vi "EL2008.vi"(8 "error in (no error)":errorcluster, 11 "EL2008 Channels":T1) -> (0 "error out":errorcluster, 3 "Read Status":bool[](array[boolean]), 7 "Write Status":bool[](array[boolean]))   [LabVIEW 2022 SP3, in "IO_Library.lvlib"]
doc: "VI implementing the EL2008.\n\nBlock reads and writes to a terminal.\n\nTo use, modify the constant string entering the ADS Init block with your string (created with the ADS Path Helper)."
uses:
  IO_Library.lvlib
  TypeDefs/EL2008Outputs.ctl
  ADS/ADS_Library.lvlib
panel:
  out "EL2008 Wc State":variant[](array[variant])
  out "bHasMatched":bool[](array[boolean])
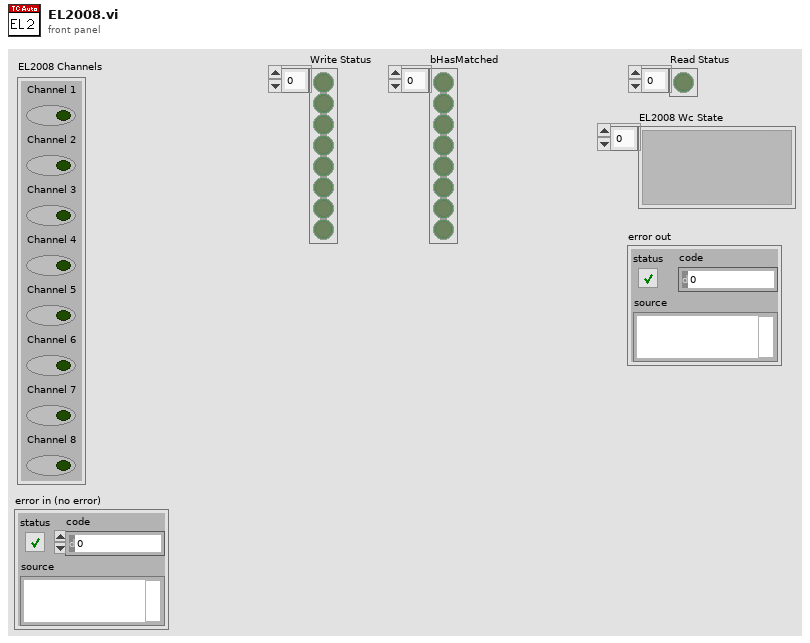
[diagram p1: front panel]
types:
  T1 = typedef "IO_Library.lvlib/EL2008Outputs.ctl" = cluster{"Channel 1":bool, "Channel 2":bool, "Channel 3":bool, "Channel 4":bool, "Channel 5":bool, "Channel 6":bool, "Channel 7":bool, "Channel 8":bool}
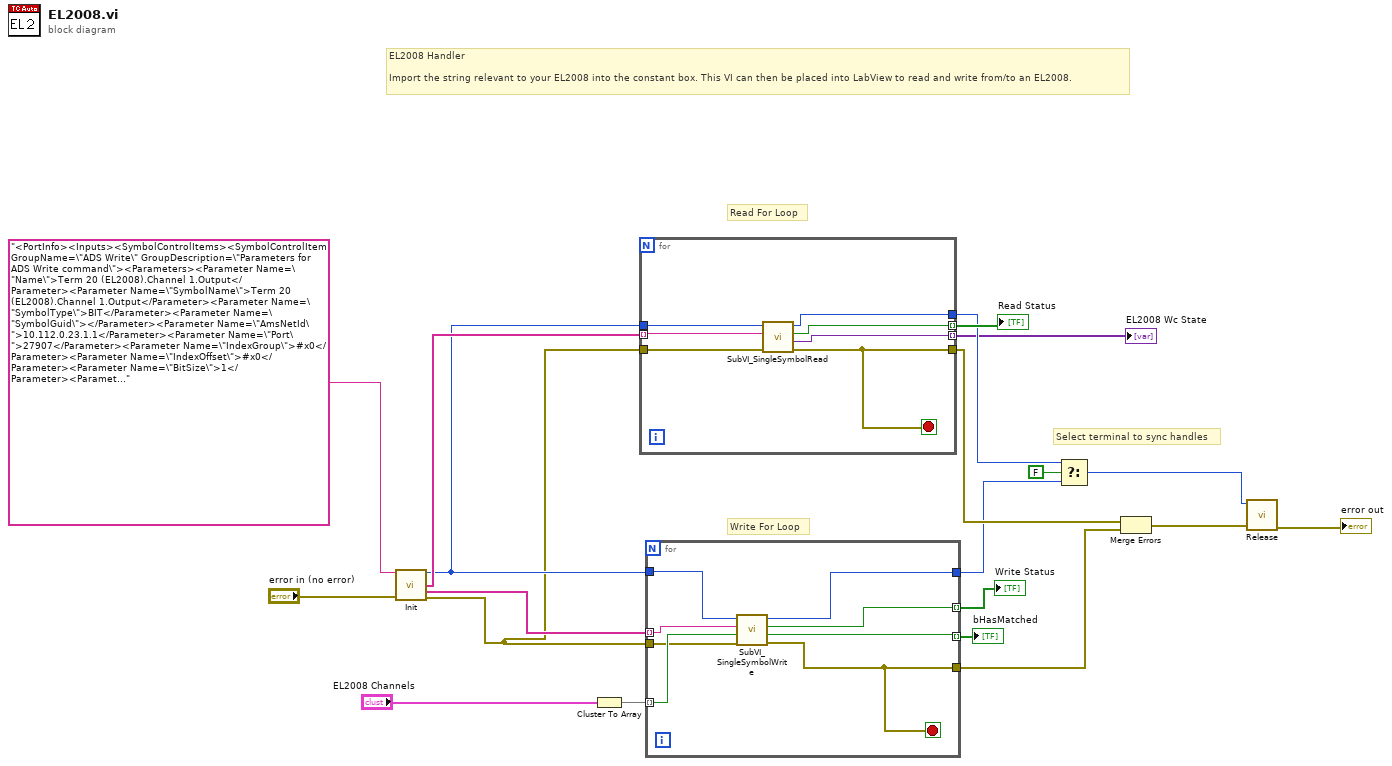
[diagram p0: block diagram]
diagram:
  # "EL2008 Handler\n\nImport the string relevant to your EL2008 into the constant box. This VI can then be placed into LabView to read and write from/to an EL2008."
  # "Select terminal to sync handles"
  # "Read For Loop"
  # "Write For Loop"
  n1 = call <userlib>:"Init.vi"("XMLDescription"="<PortInfo><Inputs><SymbolControlItems><SymbolControlItem GroupName=\"ADS Write\" GroupDescription=\"Parameters for ADS Write command\"><Parameters><Parameter Name=\"Name\">Term 20 (EL2008).Channel 1.Output</Parameter><Parameter Name=\"SymbolName\">Term 20 (EL2008).Channel 1.Output</Parameter><Parameter Name=\"SymbolType\">BIT</Parameter><Parameter Name=\"SymbolGuid\"></Parameter><Parameter Name=\"AmsNetId\">10.112.0.23.1.1</Parameter><Parameter Name=\"Port\">27907</Parameter><Parameter Name=\"IndexGroup\">#x0</Parameter><Parameter Name=\"IndexOffset\">#x0</Parameter><Parameter Name=\"BitSize\">1</Parameter><Parameter Name=\"CycleTime [ms]\">10</Parameter><Parameter Name=\"Timeout [ms]\">1000</Parameter></Parameters></SymbolControlItem><SymbolControlItem GroupName=\"ADS Write\" GroupDescription=\"Parameters for ADS Write command\"><Parameters><Parameter Name=\"Name\">Term 20 (EL2008).Channel 2.Output</Parameter><Parameter Name=\"SymbolName\">Term 20 (EL2008).Channel 2.Output</Parameter><Parameter Name=\"SymbolType\">BIT</Parameter><Parameter Name=\"SymbolGuid\"></Parameter><Parameter Name=\"AmsNetId\">10.112.0.23.1.1</Parameter><Parameter Name=\"Port\">27907</Parameter><Parameter Name=\"IndexGroup\">#x0</Parameter><Parameter Name=\"IndexOffset\">#x0</Parameter><Parameter Name=\"BitSize\">1</Parameter><Parameter Name=\"CycleTime [ms]\">10</Parameter><Parameter Name=\"Timeout [ms]\">1000</Parameter></Parameters></SymbolControlItem><SymbolControlItem GroupName=\"ADS Write\" GroupDescription=\"Parameters for ADS Write command\"><Parameters><Parameter Name=\"Name\">Term 20 (EL2008).Channel 3.Output</Parameter><Parameter Name=\"SymbolName\">Term 20 (EL2008).Channel 3.Output</Parameter><Parameter Name=\"SymbolType\">BIT</Parameter><Parameter Name=\"SymbolGuid\"></Parameter><Parameter Name=\"AmsNetId\">10.112.0.23.1.1</Parameter><Parameter Name=\"Port\">27907</Parameter><Parameter Name=\"IndexGroup\">#x0</Parameter><Parameter Name=\"IndexOffset\">#x0</Parameter><Parameter Name=\"BitSize\">1</Parameter><Parameter Name=\"CycleTime [ms]\">10</Parameter><Parameter Name=\"Timeout [ms]\">1000</Parameter></Parameters></SymbolControlItem><SymbolControlItem GroupName=\"ADS Write\" GroupDescription=\"Parameters for ADS Write command\"><Parameters><Parameter Name=\"Name\">Term 20 (EL2008).Channel 4.Output</Parameter><Parameter Name=\"SymbolName\">Term 20 (EL2008).Channel 4.Output</Parameter><Parameter Name=\"SymbolType\">BIT</Parameter><Parameter Name=\"SymbolGuid\"></Parameter><Parameter Name=\"AmsNetId\">10.112.0.23.1.1</Parameter><Parameter Name=\"Port\">27907</Parameter><Parameter Name=\"IndexGroup\">#x0</Parameter><Parameter Name=\"IndexOffset\">#x0</Parameter><Parameter Name=\"BitSize\">1</Parameter><Parameter Name=\"CycleTime [ms]\">10</Parameter><Parameter Name=\"Timeout [ms]\">1000</Parameter></Parameters></SymbolControlItem><SymbolControlItem GroupName=\"ADS Write\" GroupDescription=\"Parameters for ADS Write command\"><Parameters><Parameter Name=\"Name\">Term 20 (EL2008).Channel 5.Output</Parameter><Parameter Name=\"SymbolName\">Term 20 (EL2008).Channel 5.Output</Parameter><Parameter Name=\"SymbolType\">BIT</Parameter><Parameter Name=\"SymbolGuid\"></Parameter><Parameter Name=\"AmsNetId\">10.112.0.23.1.1</Parameter><Parameter Name=\"Port\">27907</Parameter><Parameter Name=\"IndexGroup\">#x0</Parameter><Parameter Name=\"IndexOffset\">#x0</Parameter><Parameter Name=\"BitSize\">1</Parameter><Parameter Name=\"CycleTime [ms]\">10</Parameter><Parameter Name=\"Timeout [ms]\">1000</Parameter></Parameters></SymbolControlItem><SymbolControlItem GroupName=\"ADS Write\" GroupDescription=\"Parameters for ADS Write command\"><Parameters><Parameter Name=\"Name\">Term 20 (EL2008).Channel 6.Output</Parameter><Parameter Name=\"SymbolName\">Term 20 (EL2008).Channel 6.Output</Parameter><Parameter Name=\"SymbolType\">BIT</Parameter><Parameter Name=\"SymbolGuid\"></Parameter><Parameter Name=\"AmsNetId\">10.112.0.23.1.1</Parameter><Parameter Name=\"Port\">27907</Parameter><Parameter Name=\"IndexGroup\">#x0</Parameter><Parameter Name=\"IndexOffset\">#x0</Parameter><Parameter Name=\"BitSize\">1</Parameter><Parameter Name=\"CycleTime [ms]\">10</Parameter><Parameter Name=\"Timeout [ms]\">1000</Parameter></Parameters></SymbolControlItem><SymbolControlItem GroupName=\"ADS Write\" GroupDescription=\"Parameters for ADS Write command\"><Parameters><Parameter Name=\"Name\">Term 20 (EL2008).Channel 7.Output</Parameter><Parameter Name=\"SymbolName\">Term 20 (EL2008).Channel 7.Output</Parameter><Parameter Name=\"SymbolType\">BIT</Parameter><Parameter Name=\"SymbolGuid\"></Parameter><Parameter Name=\"AmsNetId\">10.112.0.23.1.1</Parameter><Parameter Name=\"Port\">27907</Parameter><Parameter Name=\"IndexGroup\">#x0</Parameter><Parameter Name=\"IndexOffset\">#x0</Parameter><Parameter Name=\"BitSize\">1</Parameter><Parameter Name=\"CycleTime [ms]\">10</Parameter><Parameter Name=\"Timeout [ms]\">1000</Parameter></Parameters></SymbolControlItem><SymbolControlItem GroupName=\"ADS Write\" GroupDescription=\"Parameters for ADS Write command\"><Parameters><Parameter Name=\"Name\">Term 20 (EL2008).Channel 8.Output</Parameter><Parameter Name=\"SymbolName\">Term 20 (EL2008).Channel 8.Output</Parameter><Parameter Name=\"SymbolType\">BIT</Parameter><Parameter Name=\"SymbolGuid\"></Parameter><Parameter Name=\"AmsNetId\">10.112.0.23.1.1</Parameter><Parameter Name=\"Port\">27907</Parameter><Parameter Name=\"IndexGroup\">#x0</Parameter><Parameter Name=\"IndexOffset\">#x0</Parameter><Parameter Name=\"BitSize\">1</Parameter><Parameter Name=\"CycleTime [ms]\">10</Parameter><Parameter Name=\"Timeout [ms]\">1000</Parameter></Parameters></SymbolControlItem></SymbolControlItems></Inputs><Outputs><SymbolControlItems><SymbolControlItem GroupName=\"ADS Read\" GroupDescription=\"Parameters for ADS Read command\"><Parameters><Parameter Name=\"Name\">Term 20 (EL2008).WcState</Parameter><Parameter Name=\"SymbolName\">Term 20 (EL2008).WcState</Parameter><Parameter Name=\"SymbolType\">BIT</Parameter><Parameter Name=\"SymbolGuid\"></Parameter><Parameter Name=\"AmsNetId\">10.112.0.23.1.1</Parameter><Parameter Name=\"Port\">27907</Parameter><Parameter Name=\"IndexGroup\">#x0</Parameter><Parameter Name=\"IndexOffset\">#x0</Parameter><Parameter Name=\"BitSize\">1</Parameter><Parameter Name=\"CycleTime [ms]\">10</Parameter><Parameter Name=\"Transmode\">3</Parameter><Parameter Name=\"Timeout [ms]\">1000</Parameter><Parameter Name=\"TCBufferSize [Samples]\">10</Parameter><Parameter Name=\"LVBufferSize [Samples]\">50</Parameter><Parameter Name=\"Expected min delay [ms]\">500</Parameter></Parameters></SymbolControlItem></SymbolControlItems></Outputs></PortInfo>", "error in (no error)"="error in (no error)") -> ("Handle"=w12:u32, "ReadGrpSymbols"=w13:string[], "WriteGrpSymbols"=w16:string[], "error out"=w11:errorcluster)  [unwired: 9 in, 1 out]
  n2 = Cluster To Array(cluster="EL2008 Channels") -> (array=w17:bool[])
  n3 = for {
    tunnel: w13 -> [w27] mode=indexing
    tunnel: w12 -> [w26]
    tunnel: w11 -> [w25]
    tunnel: [w24] -> w9
    tunnel: [w22] -> w7 mode=indexing
    tunnel: [w23] -> w1 mode=indexing
    tunnel: [w21] -> w4
    stop <- w24 stop-if-true
    n4 = call "SubVI_SingleSymbolRead.vi"("error in (no error)"=w25, "SymbolName"=w27, "Handle In"=w26) -> ("error out"=w24:errorcluster, "RData"=w23:variant, "Read status?"=w22:bool, "Handle Out"=w21:u32)  [unwired: 5 in]
  }
  "Read Status" <- w7
  "EL2008 Wc State" <- w1
  n5 = for {
    tunnel: w17 -> [w33] mode=indexing
    tunnel: w16 -> [w34] mode=indexing
    tunnel: w11 -> [w32]
    tunnel: w12 -> [w35]
    tunnel: [w28] -> w10
    tunnel: [w30] -> w14 mode=indexing
    tunnel: [w31] -> w15 mode=indexing
    tunnel: [w29] -> w5
    stop <- w28 stop-if-true
    n6 = call "SubVI_SingleSymbolWrite.vi"("error in"=w32, "WData"=w33, "SymbolName"=w34, "Handle In"=w35) -> ("error out"=w28:errorcluster, "bHasMatched"=w30:bool, "Write Status"=w31:bool, "Handle Out"=w29:u32)  [unwired: 4 in]
  }
  "bHasMatched" <- w14
  "Write Status" <- w15
  n7 = Select(t=w4, s=FALSE, f=w5) -> (s? t:f=w2:u32)
  n8 = Merge Errors(w9, w10) -> (w8:errorcluster)
  n9 = call <userlib>:"Release.vi"("Handle"=w2, "error in (no error)"=w8) -> ("error out"=→"error out":errorcluster)  [unwired: 13 in]
